vi "Get 1D Array Image Index and Length.vi"(10 "# Image":u32, 11 "Series Graph in":refnum<class "Graph with Series View.lvclass">) -> (1 "Image Length":u32, 2 "Image Index":u32, 3 "Series Graph out":refnum<class "Graph with Series View.lvclass">)   [LabVIEW 2023, in "Graph with Series View.lvclass"]
uses:
  Graph with Series View.lvclass
  Base Graph/Base Graph.lvclass
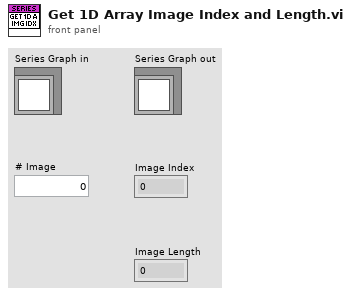
[diagram p1: front panel]
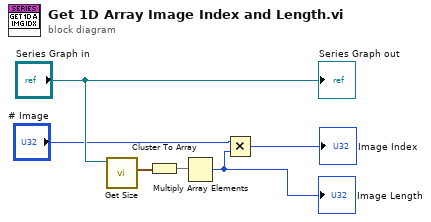
[diagram p0: block diagram]
diagram:
  n1 = call "Get Size.vi"("Base Graph in"="Series Graph in") -> ("Size"=w1:cluster{"Height":u32, "Width":u32})  [unwired: 9 in, 1 out]
  n2 = Cluster To Array(cluster=w1) -> (array=w2:u32[])
  n3 = Multiply Array Elements(1:w2) -> (0:w3:u32)
  "Image Length" <- w3
  n4 = Multiply(x="# Image", y=w3) -> (x*y=→"Image Index":u32)
  "Series Graph out" <- "Series Graph in"
